vi "HumanSetReverse.vi"(11 "Reverse":bool) -> ()   [LabVIEW 2023]
uses:
  HumanGlobal.vi
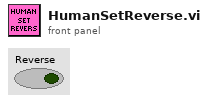
[diagram p1: front panel]
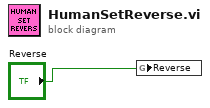
[diagram p0: block diagram]
diagram:
  n1 = global write "HumanGlobal.vi" "Reverse"("Reverse") -> ()
